vi "Publish Forward Trim.vi"(11 "Forward Trim":T1) -> ()   [LabVIEW 2016]
uses:
  <vilib>/Rock Robotics/Network Tables/NT Write Boolean.vi
  <vilib>/Rock Robotics/Network Tables/NT Write Number.vi
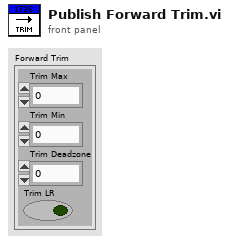
[diagram p1: front panel]
types:
  T1 = cluster{"Trim Max":dbl, "Trim Min":dbl, "Trim Deadzone":dbl, "Trim LR":bool}
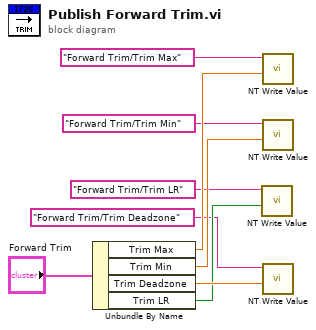
[diagram p0: block diagram]
diagram:
  n1 = Unbundle By Name("Forward Trim") -> ("Trim Max"=w9:dbl, "Trim Min"=w8:dbl, "Trim Deadzone"=w7:dbl, "Trim LR"=w6:bool)
  n2 = call-poly <vilib>:"NT Write Value.vi"("Boolean"=w6, "Name"="Forward Trim/Trim LR") -> ()  [unwired: 9 in, 1 out]
  n3 = call-poly <vilib>:"NT Write Value.vi"("Numeric"=w9, "Name"="Forward Trim/Trim Max") -> ()  [unwired: 9 in, 1 out]
  n4 = call-poly <vilib>:"NT Write Value.vi"("Numeric"=w8, "Name"="Forward Trim/Trim Min") -> ()  [unwired: 9 in, 1 out]
  n5 = call-poly <vilib>:"NT Write Value.vi"("Numeric"=w7, "Name"="Forward Trim/Trim Deadzone") -> ()  [unwired: 9 in, 1 out]
